vi "ActorCoreMassageEvent.vi"(8 "error in (no error)":errorcluster, 10 "ActorCoreEventMassage":string, 11 "UserManagement in":refnum<class "UserManagement.lvclass">) -> (0 "error out":errorcluster, 3 "UserManagement out":refnum<class "UserManagement.lvclass">)   [LabVIEW 2019, in "UserManagement.lvlib" / "UserManagement.lvclass"]
uses:
  UserManagement.lvclass
  UserManagement.lvclass/UserManagement.ctl
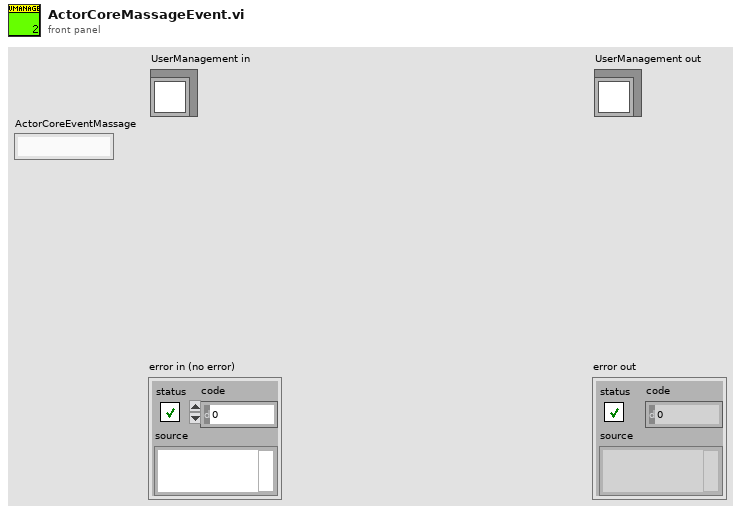
[diagram p1: front panel]
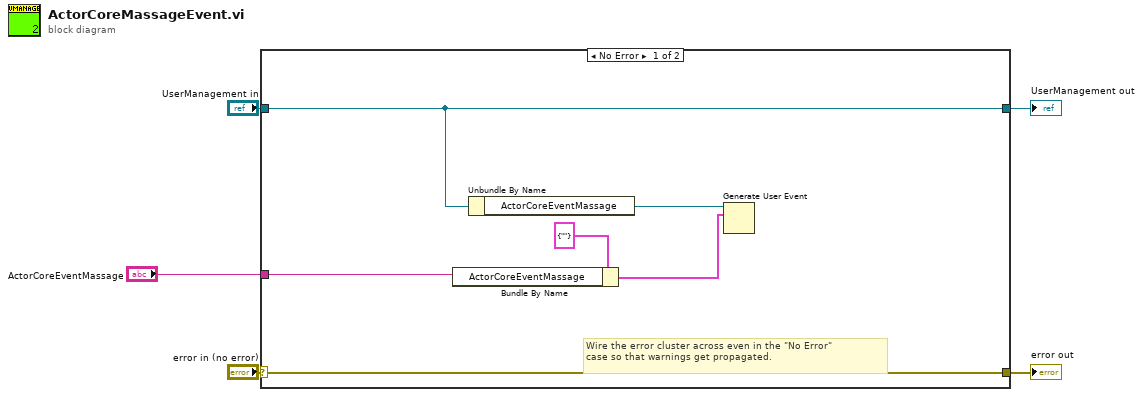
[diagram p0: block diagram]
diagram:
  n1 = case shown="No Error" "error in (no error)" {
    selector: "error in (no error)" -> [w11 w13]
    tunnel: [w11 w13] -> w4
    tunnel: [w10 w12] -> w2
    tunnel: "UserManagement in" -> [w10 w12]
    tunnel: "ActorCoreEventMassage" -> [w6 _]
    frame No Error {
      # "Wire the error cluster across even in the \"No Error\"\ncase so that warnings get propagated."
      n2 = Bundle By Name(cluster=cluster{"ActorCoreEventMassage":string} {"ActorCoreEventMassage"=""} ("event data"), "ActorCoreEventMassage"=w6) -> (w7:cluster{"ActorCoreEventMassage":string})
      n3 = Unbundle By Name(w10) -> ("ActorCoreEventMassage"=w9:refnum<user-event>)
      n4 = Generate User Event(user event=w9, event data cluster=w7) -> ()  [unwired: 2 in, 2 out]
    }
    frame Error {
    }
  }
  "error out" <- w4
  "UserManagement out" <- w2
